vi "Log.vi"(8 "Error in (no error)":errorcluster, 10 "Log in":T1 {"Priority" items=["EMERGENCY", "ALERT", "CRITICAL", "ERROR", "WARNING", "NOTICE", "INFO", "DEBUG"]}, 11 "Log in":refnum<class "Log.lvclass">) -> (0 "Error out":errorcluster, 3 "Log out":refnum<class "Log.lvclass">)   [LabVIEW 2011, in "Log.lvclass"]
uses:
  Log.lvclass
  LogCluster.ctl
  PrioritiesRing.ctl
  Log.lvclass/Log.ctl
  Filter/LogFilterInterface/LogFilterInterface.lvclass
  Writer/LogWriterInterface/LogWriterInterface.lvclass
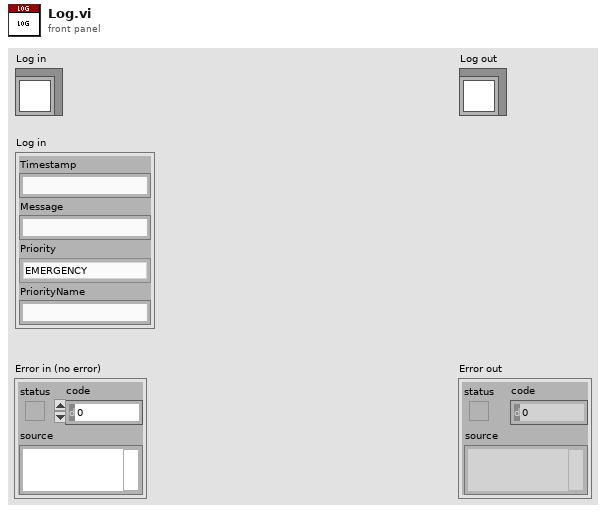
[diagram p1: front panel]
types:
  T1 = typedef "Log.lvclass/LogCluster.ctl" = cluster{"Timestamp":string, "Message":string, "Priority":T2, "PriorityName":string}
  T2 = typedef "Log.lvclass/PrioritiesRing.ctl" = u32
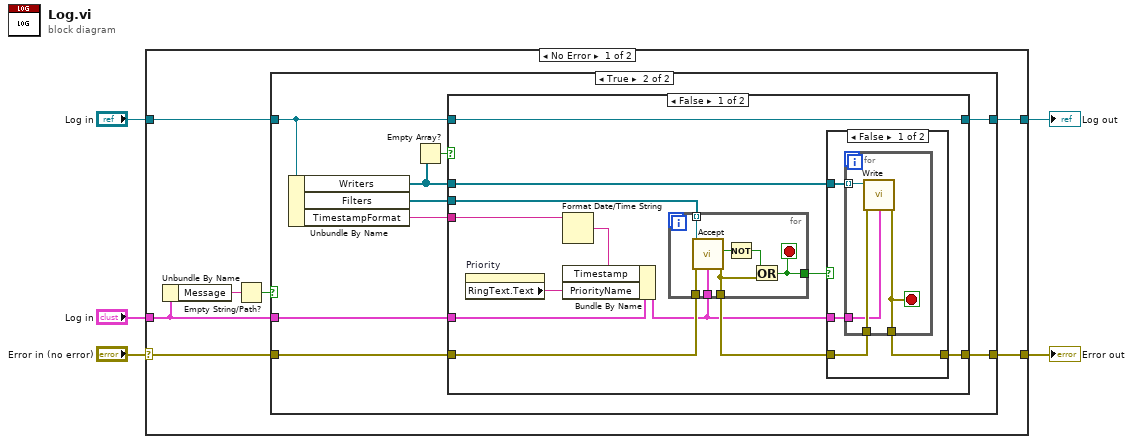
[diagram p0: block diagram]
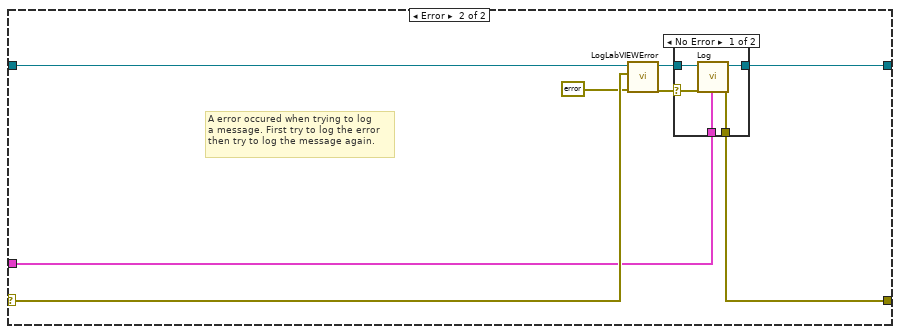
[diagram p5: hidden frame]
diagram:
  n1 = case shown="No Error" "Error in (no error)" {
    selector: "Error in (no error)" -> [w10 w61]
    tunnel: [w9 w56] -> w4
    tunnel: [w11 w57] -> w2
    tunnel: "Log in" -> [w12 w60]
    tunnel: "Log in" -> [w8 w54]
    frame No Error {
      n2 = Unbundle By Name(w8) -> ("Message"=w6:string)
      n3 = Empty String/Path?(string/path=w6) -> (empty?=w7:bool)
      n4 = case shown="True" w7 {
        tunnel: w12 -> [w14 w22]
        tunnel: [w14 w20] -> w11
        tunnel: w10 -> [w13 w18]
        tunnel: [w13 w17] -> w9
        tunnel: w8 -> [_ w15]
        frame False {
          # "Error, no message"
        }
        frame True {
          n5 = Unbundle By Name(w22) -> ("Writers"=w19:refnum<class "LogWriterInterface.lvclass">[], "Filters"=w21:refnum<class "LogFilterInterface.lvclass">[], "TimestampFormat"=w16:string)
          n6 = Empty Array?(array=w19) -> (empty?=w23:bool)
          n7 = case shown="False" w23 {
            tunnel: w22 -> [w32 w53]
            tunnel: w21 -> [w35 _]
            tunnel: w16 -> [w34 _]
            tunnel: w19 -> [w33 _]
            tunnel: [w32 w53] -> w20
            tunnel: w18 -> [w30 w52]
            tunnel: [w31 w52] -> w17
            tunnel: w15 -> [w25 _]
            frame False {
              n8 = property on="Priority" class="Ring (strict)"() -> ("RingText.Text"=w24:string)  [unwired: 2 in, 2 out]
              n9 = Format Date/Time String(time format string (%c)=w34) -> (date/time string=w29:string)  [unwired: 2 in]
              n10 = Bundle By Name(cluster=w25, "Timestamp"=w29, "PriorityName"=w24) -> (w26:T1)
              n11 = for {
                tunnel: w26 -> [w46]
                tunnel: w35 -> [w51] mode=indexing
                tunnel: w30 -> [w50]
                tunnel: [w48] -> w28
                tunnel: [w47] -> w27
                stop <- w47 stop-if-true
                n12 = call-dynamic "Accept.vi"("Error in (no error)"=w50, "Log in"=w46, "LogFilterInterface in"=w51) -> ("Error out"=w48:errorcluster, "Accept"=w49:bool)  [unwired: 6 in, 1 out]
                n13 = Not(x=w49) -> (.not. x?=w45:bool)
                n14 = Or(x=w45, y=w48) -> (x .or. y?=w47:bool)
              }
              n15 = case shown="False" w27 {
                tunnel: w33 -> [w39 _]
                tunnel: w28 -> [w37 w44]
                tunnel: [w36 w44] -> w31
                tunnel: w26 -> [w38 _]
                frame False {
                  n16 = for {
                    tunnel: w39 -> [w43] mode=indexing
                    tunnel: w37 -> [w42]
                    tunnel: w38 -> [w41]
                    tunnel: [w40] -> w36
                    stop <- w40 stop-if-true
                    n17 = call "Write.vi"("Error in (no error)"=w42, "Log in"=w41, "LogWriterInterface in"=w43) -> ("Error out"=w40:errorcluster)  [unwired: 7 in, 1 out]
                  }
                }
                frame True {
                  # "Log message\nwas filtered"
                }
              }
            }
            frame True {
              # "Error, no writer"
            }
          }
        }
      }
    }
    frame Error {
      # "A error occured when trying to log\na message. First try to log the error \nthen try to log the message again."
      n18 = call "LogLabVIEWError.vi"("Error in (no error)"=errorcluster {"status"=FALSE, "code"=0, "source"=""}, "Error in"=w61, "Log in"=w60) -> ("Error out"=w55:errorcluster, "Log out"=w58:refnum<class "Log.lvclass">)  [unwired: 7 in]
      n19 = case shown="No Error" w55 {
        selector: w55 -> [w63 w67]
        tunnel: w58 -> [w66 w68]
        tunnel: [w65 w68] -> w57
        tunnel: [w64 w67] -> w56
        tunnel: w54 -> [w62 _]
        frame No Error {
          n20 = call "Log.vi"("Error in (no error)"=w63, 10:"Log in"=w62, 11:"Log in"=w66) -> ("Error out"=w64:errorcluster, "Log out"=w65:refnum<class "Log.lvclass">)  [unwired: 7 in]
        }
        frame Error {
        }
      }
    }
  }
  "Error out" <- w4
  "Log out" <- w2
